vi "CLD 14 Timer Application Exercise.vi"() -> ()   [LabVIEW 2009]
panel:
  out "Time Target (S)":dbl
  out "Elapsed Time (S)":dbl
  in  "Stop":bool
  in  "Pause":bool
  in  "cancel":bool
  in  "Start":bool
  in  "Error In":errorcluster
  out "Error Out":errorcluster
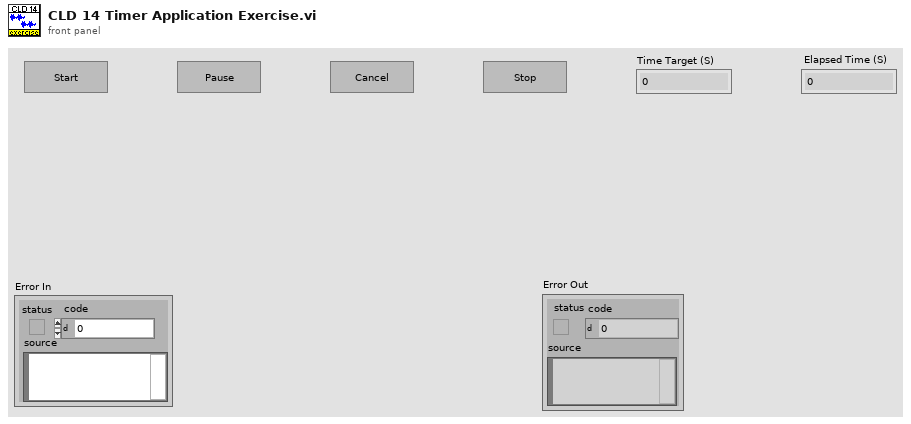
[diagram p1: front panel]
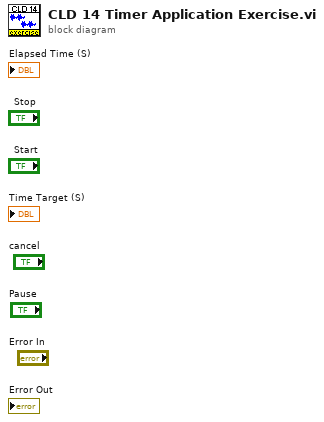
[diagram p0: block diagram]
diagram:
